vi "DI init.vi"(10 "N_param":i32) -> (0 "error":errorcluster, 3 "DI":T1)   [LabVIEW 2019, in "Inputs.lvlib"]
uses:
  Inputs.lvlib
  Ctl/DI.ctl
  Ctl/DI short.ctl
  Ctl/Parameter State.ctl
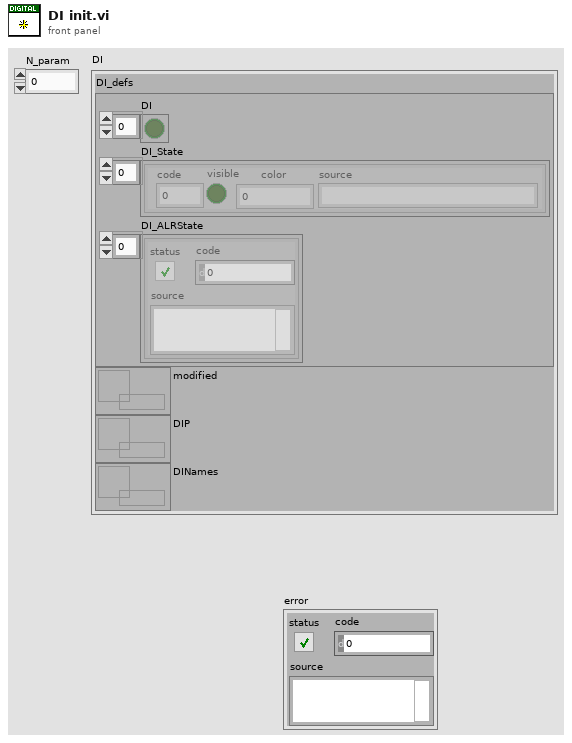
[diagram p1: front panel]
types:
  T1 = typedef "Inputs.lvlib/DI.ctl" = cluster{"DI_defs":T2, "modified":refnum<data-value>, "DIP":refnum<data-value>, "DINames":refnum<data-value>}
  T2 = typedef "Inputs.lvlib/DI short.ctl" = cluster{"DI":bool[], "DI_State":T3[], "DI_ALRState":errorcluster[]}
  T3 = typedef "Inputs.lvlib/Parameter State.ctl" = cluster{"code":i32, "visible":bool, "color":u32, "source":string}
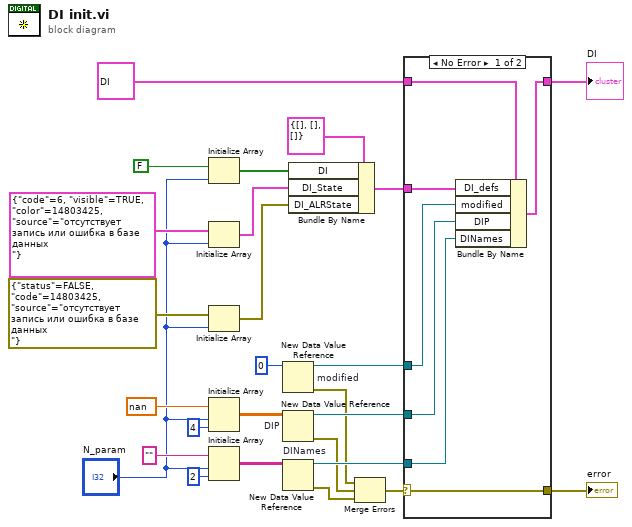
[diagram p0: block diagram]
diagram:
  n1 = Initialize Array(FALSE, "N_param") -> (w24:bool[])
  n2 = Initialize Array(T3 {"code"=6, "visible"=TRUE, "color"=14803425, "source"="отсутствует запись или ошибка в базе данных                                                                                    "} ("STATE"), "N_param") -> (w23:T3[])
  n3 = Initialize Array(errorcluster {"status"=FALSE, "code"=14803425, "source"="отсутствует запись или ошибка в базе данных                                                                                    "} ("ALRSTATE"), "N_param") -> (w22:errorcluster[])
  n4 = Initialize Array(nan ("DIP"), "N_param", 4 ("dimension size")) -> (w8:dbl[][])
  n5 = Initialize Array("" ("AINames"), "N_param", 2 ("dimension size")) -> (w16:string[][])
  n6 = New Data Value Reference "modified"(data value=u8 0 ("modified")) -> (data value reference=w6:refnum<data-value>, error out=w4:errorcluster)  [unwired: 1 in]
  n7 = New Data Value Reference "DIP"(data value=w8) -> (data value reference=w7:refnum<data-value>, error out=w3:errorcluster)  [unwired: 1 in]
  n8 = New Data Value Reference "DINames"(data value=w16) -> (data value reference=w15:refnum<data-value>, error out=w2:errorcluster)  [unwired: 1 in]
  n9 = Bundle By Name(cluster=T2 {"DI"=[], "DI_State"=[], "DI_ALRState"=[]} ("DI_defs"), "DI"=w24, "DI_State"=w23, "DI_ALRState"=w22) -> (w12:T2)
  n10 = Merge Errors(w4, w3, w2) -> (w5:errorcluster)
  n11 = case shown="No Error" w5 {
    selector: w5 -> [w30 w35]
    tunnel: w7 -> [w28 _]
    tunnel: w15 -> [w29 _]
    tunnel: [w30 w35] -> w13
    tunnel: w12 -> [w32 _]
    tunnel: T1 {"DI_defs"={"DI"=[], "DI_State"=[], "DI_ALRState"=[]}, "modified"=refnum, "DIP"=refnum, "DINames"=refnum} ("DI") -> [w33 w34]
    tunnel: [w31 w34] -> w10
    tunnel: w6 -> [w27 _]
    frame No Error {
      n12 = Bundle By Name(cluster=w33, "DI_defs"=w32, "modified"=w27, "DIP"=w28, "DINames"=w29) -> (w31:T1)
    }
    frame Error {
    }
  }
  "error" <- w13
  "DI" <- w10
